vi "SetGeometry.vi"(8 "error in (no error)":errorcluster, 10 "Geometry":refnum<vi>[](array[refnum]), 11 "reference in":refnum<class "SceneObject.lvclass">) -> (0 "error out":errorcluster, 3 "reference out":refnum<class "SceneObject.lvclass">)   [LabVIEW 2010, in "RenderBase.lvlib" / "SceneObject.lvclass"]
uses:
  SceneObject.lvclass
  SceneObject.lvclass/SceneObject.ctl
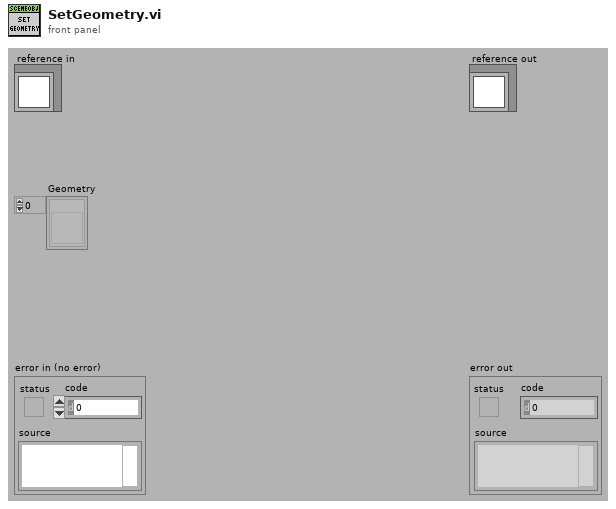
[diagram p1: front panel]
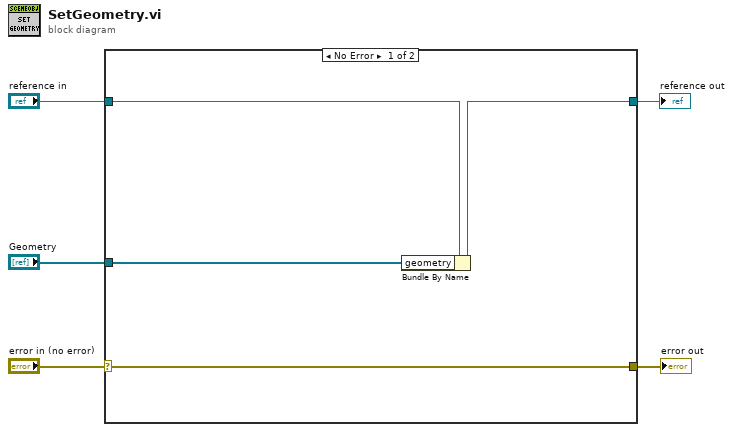
[diagram p0: block diagram]
diagram:
  n1 = case shown="No Error" "error in (no error)" {
    selector: "error in (no error)" -> [w7 w11]
    tunnel: [w7 w11] -> w4
    tunnel: [w8 w10] -> w2
    tunnel: "reference in" -> [w9 w10]
    tunnel: "Geometry" -> [w6 _]
    frame No Error {
      n2 = Bundle By Name(cluster=w9, "geometry"=w6) -> (w8:refnum<class "SceneObject.lvclass">)
    }
    frame Error {
    }
  }
  "error out" <- w4
  "reference out" <- w2
